vi "Shared data buffer.vi"(8 "command":T3, 9 "Shared data names (unit) in":string[](array[string]), 10 "Data from local sources in":T1 {"Sensor array"."scaled" format="%.2f"; "Sensor array"."voltage" format="%.4f"; "Time" format="%<%I:%M:%S%2u %p\n%m/%d/%Y>T"}, 11 "Data from shared sources in":T1 {"Sensor array"."scaled" format="%.2f"; "Sensor array"."voltage" format="%.4f"; "Time" format="%<%I:%M:%S%2u %p\n%m/%d/%Y>T"}) -> (1 "Shared data names (unit) out":string[](array[string]), 2 "Data from merged sources out":T1 {"Sensor array"."scaled" format="%.2f"; "Sensor array"."voltage" format="%.4f"; "Time" format="%<%I:%M:%S%2u %p\n%m/%d/%Y>T"}, 3 "Data from shared sources out":T1 {"Sensor array"."scaled" format="%.2f"; "Sensor array"."voltage" format="%.4f"; "Time" format="%<%I:%M:%S%2u %p\n%m/%d/%Y>T"})   [LabVIEW 2015]
uses:
  buffer.ctl
  TCP DAQ/Sensor data.ctl
  DAQ configuration/sensor cluster.ctl
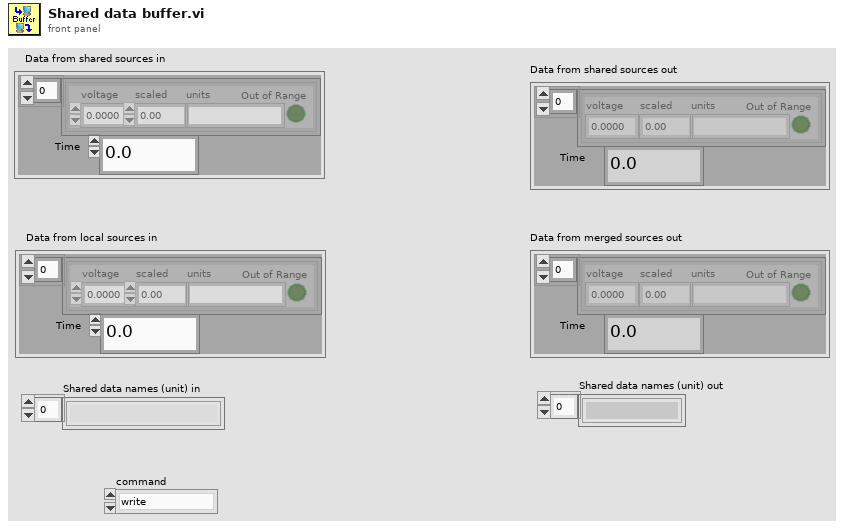
[diagram p1: front panel]
types:
  T1 = typedef "Sensor data.ctl" = cluster{" Sensor array":T2[], "Time":dbl}
  T2 = typedef "sensor cluster.ctl" = cluster{"voltage":sgl, "scaled":sgl, "units":string, "Out of Range":bool}
  T3 = typedef "buffer.ctl" = enum16{"write", "read", "read merge"}
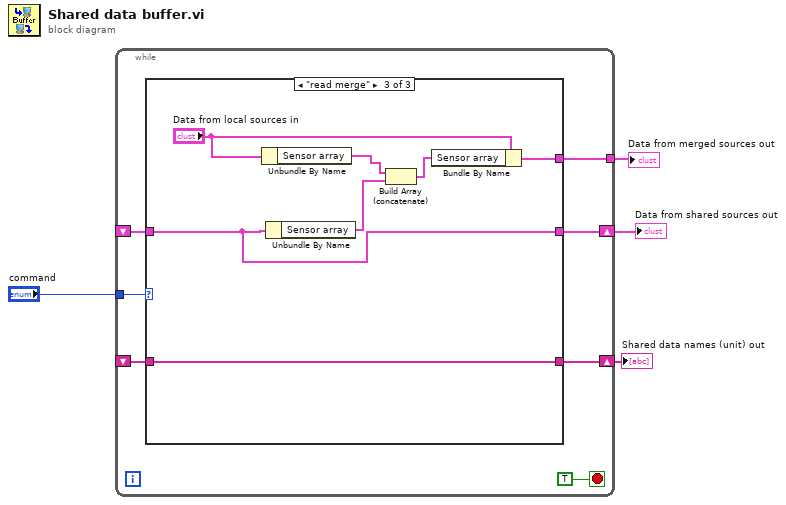
[diagram p0: block diagram]
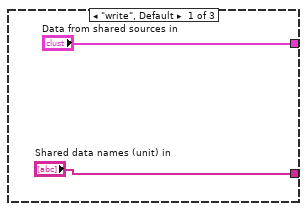
[diagram p2: hidden frame]
diagram:
  n1 = while {
    tunnel: "command" -> [w10]
    shift-right: [w9] -> w3
    shift-left: _ -> [w8]
    tunnel: [w7] -> w2
    shift-right: [w6] -> w1
    shift-left: _ -> [w5]
    stop <- TRUE stop-if-true
    n2 = case shown="\"read merge\"" w10 {
      tunnel: ["Data from shared sources in" w15 w17] -> w9
      tunnel: w8 -> [_ w15 w17]
      tunnel: [_ _ w18] -> w7
      tunnel: ["Shared data names (unit) in" w14 w16] -> w6
      tunnel: w5 -> [_ w14 w16]
      frame "write", Default {
      }
      frame "read" {
      }
      frame "read merge" {
        n3 = Unbundle By Name("Data from local sources in") -> ("Sensor array"=w22:T2[])
        n4 = Unbundle By Name(w17) -> ("Sensor array"=w21:T2[])
        n5 = Build Array (concatenate)(w22, w21) -> (w19:T2[])
        n6 = Bundle By Name(cluster="Data from local sources in", "Sensor array"=w19) -> (w18:T1)
      }
    }
  }
  "Data from shared sources out" <- w3
  "Data from merged sources out" <- w2
  "Shared data names (unit) out" <- w1
